vi "Main Page.vi"(8 "error in":errorcluster, 11 "Node Ptr":T1 format="%.0x") -> (0 "error out":errorcluster)   [LabVIEW 2026, in "Template System Explorer.lvlib"]
uses:
  <vilib>/NI VeriStand/Custom Device API/Custom Device Item Ref.ctl
  NationalInstruments.VeriStand.SystemDefinitionAPI
  Template System Explorer.lvlib
  <vilib>/NI VeriStand/Custom Device API/Custom Device API.lvlib
  C:/Program Files/National Instruments/VeriStand 2026/NationalInstruments.VeriStand.Controls.dll
  Program Files/National Instruments/VeriStand 2026/NationalInstruments.VeriStand.Controls.dll
panel:
  in  "PagePropertyEditor":refnum<k24>(container)
  out "Version":string
  in  "Browser":refnum<k7>(container)
  in  "Specific Header":cluster{"Section Name":string}={"Section Name"="Custom Device Item Settings"}
  in  "General Header":cluster{"Section Name":string}={"Section Name"="General Custom Device Settings"}
  in  "Description":string
  in  "Name":string
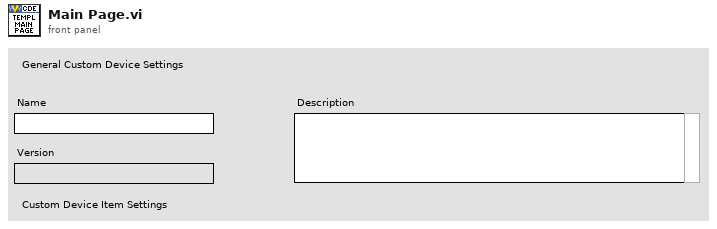
[diagram p1: front panel]
types:
  T1 = typedef "Custom Device API.lvlib/Custom Device Item Ref.ctl" = u64
  T2 = typedef "Custom Device API.lvlib/Custom Device Item Info.ctl" = cluster{"Name":string, "Is Channel":bool, "GUID":string, "Is Waveform":bool}
  T3 = typedef "Custom Device API.lvlib/Custom Device Commands.ctl" = enum16{"Default", "Item renamed", "Shutdown", "Dynamic button pressed"}
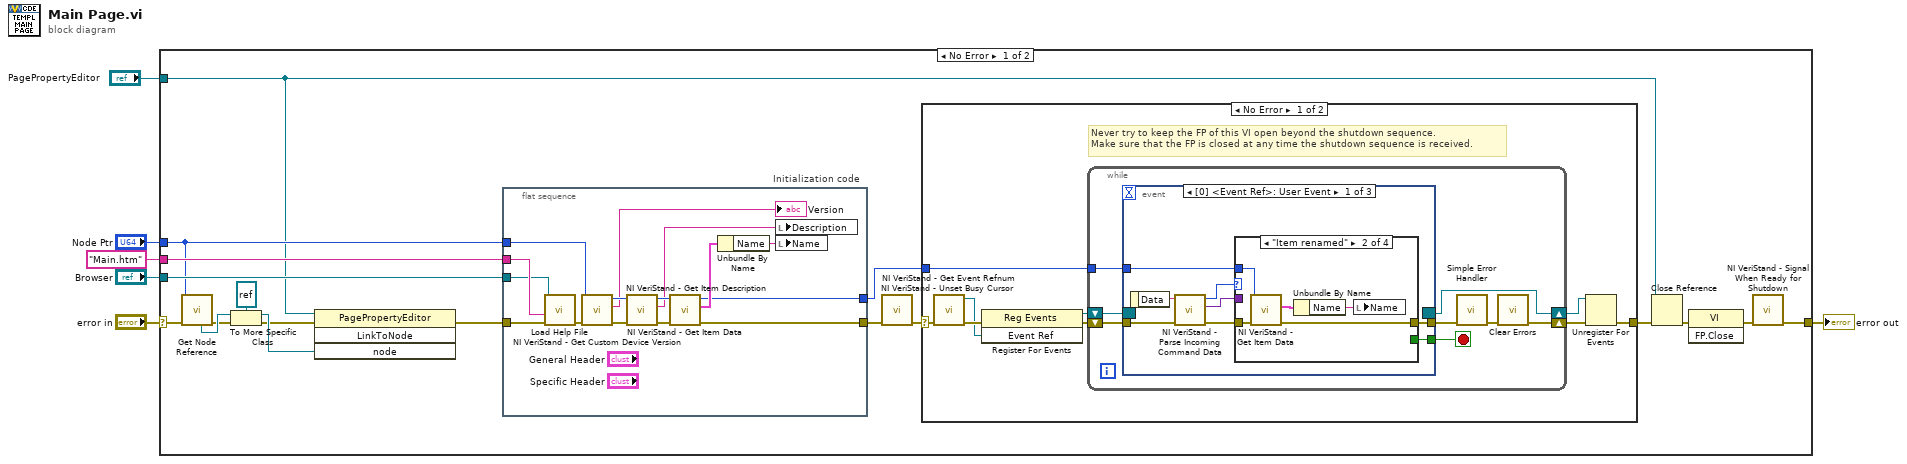
[diagram p0: block diagram]
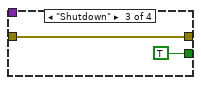
[diagram p3: hidden frame]
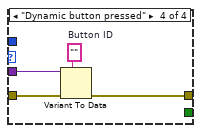
[diagram p4: hidden frame]
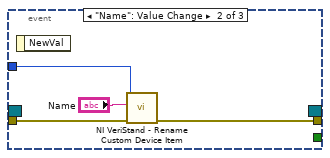
[diagram p5: hidden frame]
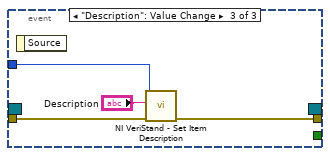
[diagram p6: hidden frame]
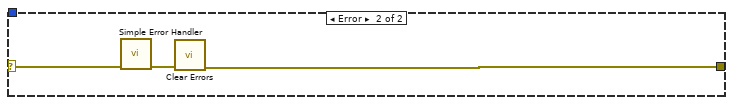
[diagram p7: hidden frame]
diagram:
  n1 = case shown="No Error" "error in" {
    selector: "error in" -> [w17 w88]
    tunnel: [w24 w88] -> w2
    tunnel: "Node Ptr" -> [w16 _]
    tunnel: "Browser" -> [w23 _]
    tunnel: "Main.htm" ("HTML File") -> [w22 _]
    tunnel: "PagePropertyEditor" -> [w12 _]
    frame No Error {
      n2 = call "Get Node Reference.vi"("error in"=w17, "Node Ptr"=w16) -> ("error out"=w8:errorcluster, "Base Node"=w11:refnum<k24>)  [unwired: 6 in, 2 out]
      n3 = To More Specific Class(target class=refnum<k24> refnum, reference=w11, error in=w8) -> (specific class reference=w9:refnum<k24>, error out=w7:errorcluster)
      n4 = invoke class="PagePropertyEditor" method="LinkToNode"(reference=w12, error in=w7, "node"=w9) -> (error out=w15:errorcluster)  [unwired: 1 in, 3 out]
      n5 = flat-sequence "Initialization code" {
        tunnel: w15 -> [w37]
        tunnel: w16 -> [w32]
        tunnel: [w35] -> w18
        tunnel: [w25] -> w19
        tunnel: w23 -> [w26]
        tunnel: w22 -> [w27]
        frame #0 {
          n6 = call "Load Help File.vi"("error in"=w37, "HTML File to Load"=w27, "Browser"=w26) -> ("error out"=w36:errorcluster)  [unwired: 8 in]
          n7 = call <vilib>:"NI VeriStand - Get Custom Device Version.vi"("error in (no error)"=w36, "Device Ref in"=w32) -> ("error out"=w38:errorcluster, "Value"=→"Version":string, "Device Ref out"=w31:T1)  [unwired: 7 in]
          n8 = call <vilib>:"NI VeriStand - Get Item Description.vi"("error in (no error)"=w38, "Item Ref in"=w31) -> ("error out"=w39:errorcluster, "Description"=w28:string, "Item Ref out"=w34:T1)  [unwired: 7 out]
          n9 = call <vilib>:"NI VeriStand - Get Item Data.vi"("error in (no error)"=w39, "Item Ref in"=w34) -> ("error out"=w35:errorcluster, "Item Info"=w33:T2, "Item Ref out"=w25:T1)  [unwired: 7 out]
          n10 = Unbundle By Name(w33) -> ("Name"=w29:string)
          n11 = local write "Description"(w28) -> ()
          n12 = local write "Name"(w29) -> ()
        }
      }
      n13 = call <vilib>:"NI VeriStand - Unset Busy Cursor.vi"("error in (no error)"=w18) -> ("error out"=w20:errorcluster)  [unwired: 10 out]
      n14 = case shown="No Error" w20 {
        selector: w20 -> [w44 w87]
        tunnel: [w46 w85] -> w14
        tunnel: w19 -> [w40 _]
        frame No Error {
          # "Never try to keep the FP of this VI open beyond the shutdown sequence.\nMake sure that the FP is closed at any time the shutdown sequence is received."
          n15 = call <vilib>:"NI VeriStand - Get Event Refnum.vi"("error in (no error)"=w44) -> ("error out"=w48:errorcluster, "Event Ref"=w42:refnum<user-event>)  [unwired: 9 out]
          n16 = register-events(error in=w48, w42) -> (reference out=w41:refnum<event-registration>, error out=w45:errorcluster)  [unwired: 1 in]
          n17 = while {
            tunnel: w40 -> [w49]
            shift-right: [w53] -> w47
            shift-left: w45 -> [w56]
            shift-right: [w52] -> w43
            shift-left: w41 -> [w51]
            stop <- w50 stop-if-true
            n18 = event shown="[0] <Event Ref>: User Event" {
              selector: w51 -> [_ _ _]
              dyn-events: [_ _ _] -> w52
              timeout: _ -> [_ _ _]
              tunnel: w56 -> [w64 w80 w84]
              tunnel: [w59 _ _] -> w50
              tunnel: [w62 w79 w83] -> w55
              tunnel: w49 -> [w58 w78 w82]
              event User Event {
                n19 = event-data() -> ("Data"=w61:string)  [unwired: 1 out]
                n20 = call <vilib>:"NI VeriStand - Parse Incoming Command Data.vi"("error in (no error)"=w64, "Incoming data"=w61) -> ("error out"=w63:errorcluster, "Outgoing data"=w57:variant, "Action"=w60:T3)  [unwired: 7 out]
                n21 = case shown="\"Item renamed\"" w60 {
                  tunnel: w63 -> [w65 w70 w72 w76]
                  tunnel: [_ _ TRUE _] -> w59
                  tunnel: [w65 w69 w72 w75] -> w62
                  tunnel: w58 -> [_ w68 _ _]
                  tunnel: w57 -> [_ _ _ w74]
                  frame "Default", Default {
                  }
                  frame "Item renamed" {
                    n22 = call <vilib>:"NI VeriStand - Get Item Data.vi"("error in (no error)"=w70, "Item Ref in"=w68) -> ("error out"=w69:errorcluster, "Item Info"=w67:T2)  [unwired: 8 out]
                    n23 = Unbundle By Name(w67) -> ("Name"=w66:string)
                    n24 = local write "Name"(w66) -> ()
                  }
                  frame "Shutdown" {
                  }
                  frame "Dynamic button pressed" {
                    w73 = ""  # Button ID
                    n25 = Variant To Data(error in=w76, type=w73, Variant=w74) -> (error out=w75:errorcluster)  [unwired: 1 out]
                  }
                }
              }
              event "Name": Value Change {
                n26 = event-data() -> ()  [unwired: 2 out]
                n27 = call <vilib>:"NI VeriStand - Rename Custom Device Item.vi"("error in (no error)"=w80, "New Name"="Name", "Item Ref in"=w78) -> ("error out"=w79:errorcluster)  [unwired: 1 in, 7 out]
              }
              event "Description": Value Change {
                n28 = event-data() -> ()  [unwired: 2 out]
                n29 = call <vilib>:"NI VeriStand - Set Item Description.vi"("error in (no error)"=w84, "Description"="Description", "Item Ref in"=w82) -> ("error out"=w83:errorcluster)  [unwired: 8 out]
              }
            }
            n30 = call <vilib>:"Simple Error Handler.vi"("error in (no error)"=w55) -> ("error out"=w54:errorcluster)  [unwired: 1 in, 7 out]
            n31 = call <vilib>:"Clear Errors.vi"("error in (no error)"=w54) -> ("error out"=w53:errorcluster)  [unwired: 1 in, 5 out]
          }
          n32 = Unregister For Events(event registration refnum=w43, error in=w47) -> (error out=w46:errorcluster)
        }
        frame Error {
          n33 = call <vilib>:"Simple Error Handler.vi"("error in (no error)"=w87) -> ("error out"=w86:errorcluster)  [unwired: 1 in, 7 out]
          n34 = call <vilib>:"Clear Errors.vi"("error in (no error)"=w86) -> ("error out"=w85:errorcluster)  [unwired: 1 in, 5 out]
        }
      }
      n35 = Close Reference(reference=w12, error in (no error)=w14) -> (error out=w13:errorcluster)
      n36 = invoke class="VI" method="FP.Close"(error in=w13) -> (error out=w21:errorcluster)  [unwired: 2 in, 2 out]
      n37 = call <vilib>:"NI VeriStand - Signal When Ready for Shutdown.vi"("error in (no error)"=w21) -> ("error out"=w24:errorcluster)  [unwired: 10 out]
    }
    frame Error {
    }
  }
  "error out" <- w2
